vi "Relink Packages.vi"(8 "error in (no error)":errorcluster, 11 "Folders to relink":string[](array[string])) -> (0 "error out":errorcluster, 1 "Done":bool, 2 "report log out":string[](array[string]), 3 "Saved Items out":T1(array[cluster]))   [LabVIEW 2020]
doc: "Relinks LabVIEW packages after files were moved, generalising Relink Package.vi from one folder to an array of folders.\n\nTwo-phase design: Phase A (discovering) opens every .lvlib/.lvclass under each folder (loading makes LabVIEW relink moved dependencies), walks their descendants and opens every loose .vi/.ctl/.vim not owned by a library. Nothing is saved in Phase A and every reference is held open across all folders (warm object cache). Libraries and items are deduplicated globally across folders and packages. Work items are collected as ONE cluster array {Folder, Name, Type String, Path, ref} - each library's own item is appended AFTER its members, so members always save before their owning library. The ref field is a variant carrying the VI or Library refnum (To Variant when collecting, Variant To Data with the class picked by Type String when saving/closing). Null-ref filtering: Get All Descendents also returns non-VI project items whose 'VI Reference' property reads back a null (0) refnum WITHOUT an error, so a descendant becomes a work item only when its Type String is 'VI' AND the VI Reference read had no error AND the refnum passes Not A Number/Path/Refnum?. A library whose open or descendant walk fails is recorded in Saved Items out (Type String 'Library', status = TRUE), its reference is closed immediately and never enters the work-item array.\n\nPhase B (saving) saves EVERY work item unconditionally - there is deliberately no dirty gate. Rationale: LabVIEW resolves moved/stale subVI paths at load WITHOUT setting the VI Modifications Bitset (measured: a VI with dead absolute linker paths read bitset = 0), so gating on the bitset skips exactly the files whose linker table needs rewriting. Unconditional saving matches VIPM behaviour. A failing save never aborts the pass - it is recorded per item in Saved Items out (status = TRUE). All references are closed after Phase B and Done becomes TRUE only after the closes complete.\n\nVI-Server polling contract: the caller sets 'Folders to relink' and error in, runs the VI, and may poll Progress Phase ('discovering' then 'saving'), Progress Total, Progress Done and Progress Item while it runs. With an empty folder array the VI finishes immediately with Done = TRUE, empty reports and no error."
uses:
  a6c5ae95-22bd-4c75-b5e1-b7ef04b7ddf2.vi
  018dfcb9-4c8e-49be-be6d-b19c84c3ecea.vi
  f1460510-d6ef-45a5-b954-0afa6c603d40.vi
  0105af62-cf63-4b41-8393-fe647030f84d.vi
  a43e3b37-a8ff-4dec-b57d-d584032e0765.vi
panel:
  out "Progress Item":string
  out "Progress Done":i32
  out "Progress Total":i32
  out "Progress Phase":string
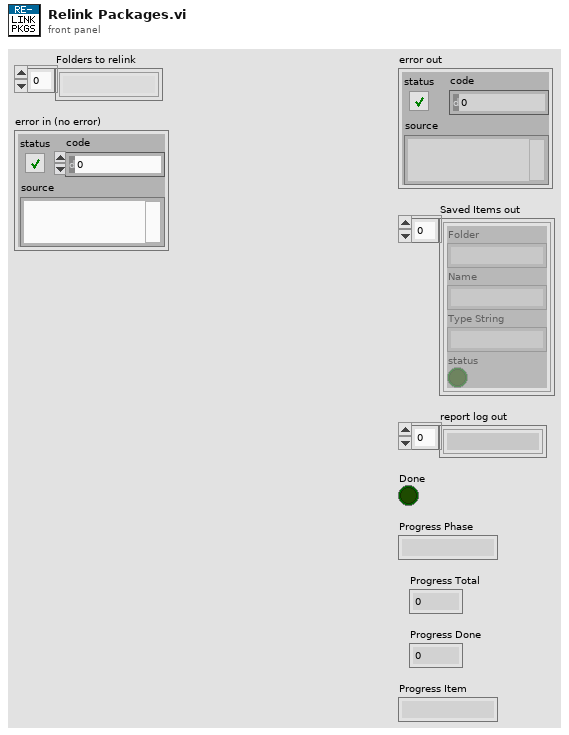
[diagram p1: front panel]
types:
  T1 = cluster{"Folder":string, "Name":string, "Type String":string, "status":bool}[]
  T2 = cluster{"Folder":string, "Name":string, "Type String":string, "Path":string, "ref":variant}[]
  T3 = cluster{"Folder":string, "Name":string, "Type String":string, "Path":string, "ref":variant}
  T4 = cluster{"Folder":string, "Name":string, "Type String":string, "status":bool}
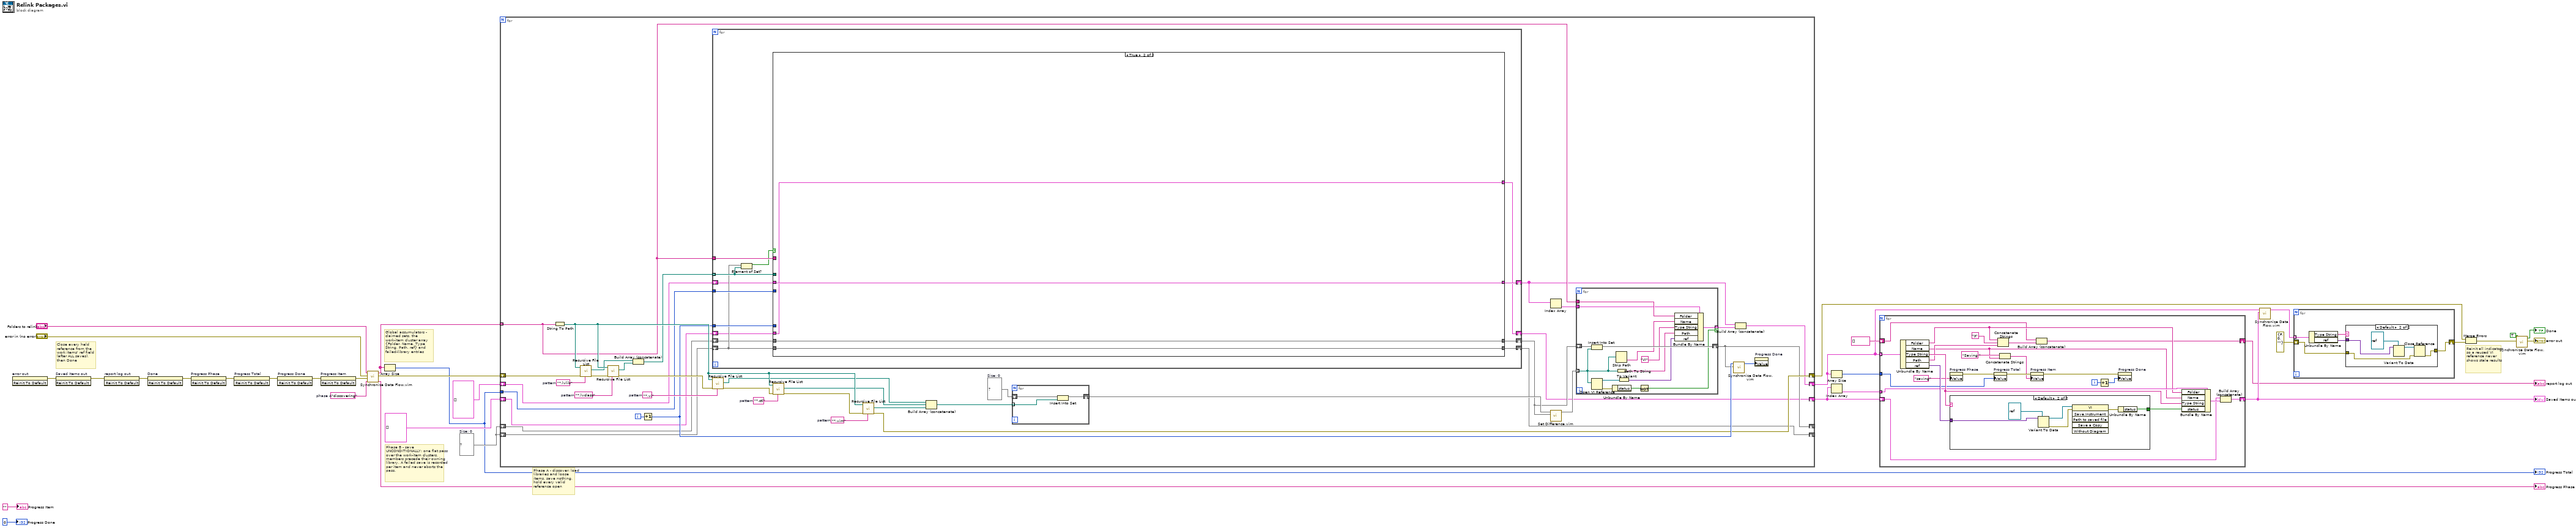
[diagram p0: block diagram]
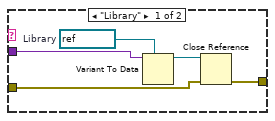
[diagram p2: hidden frame]
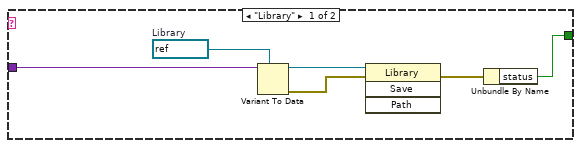
[diagram p3: hidden frame]
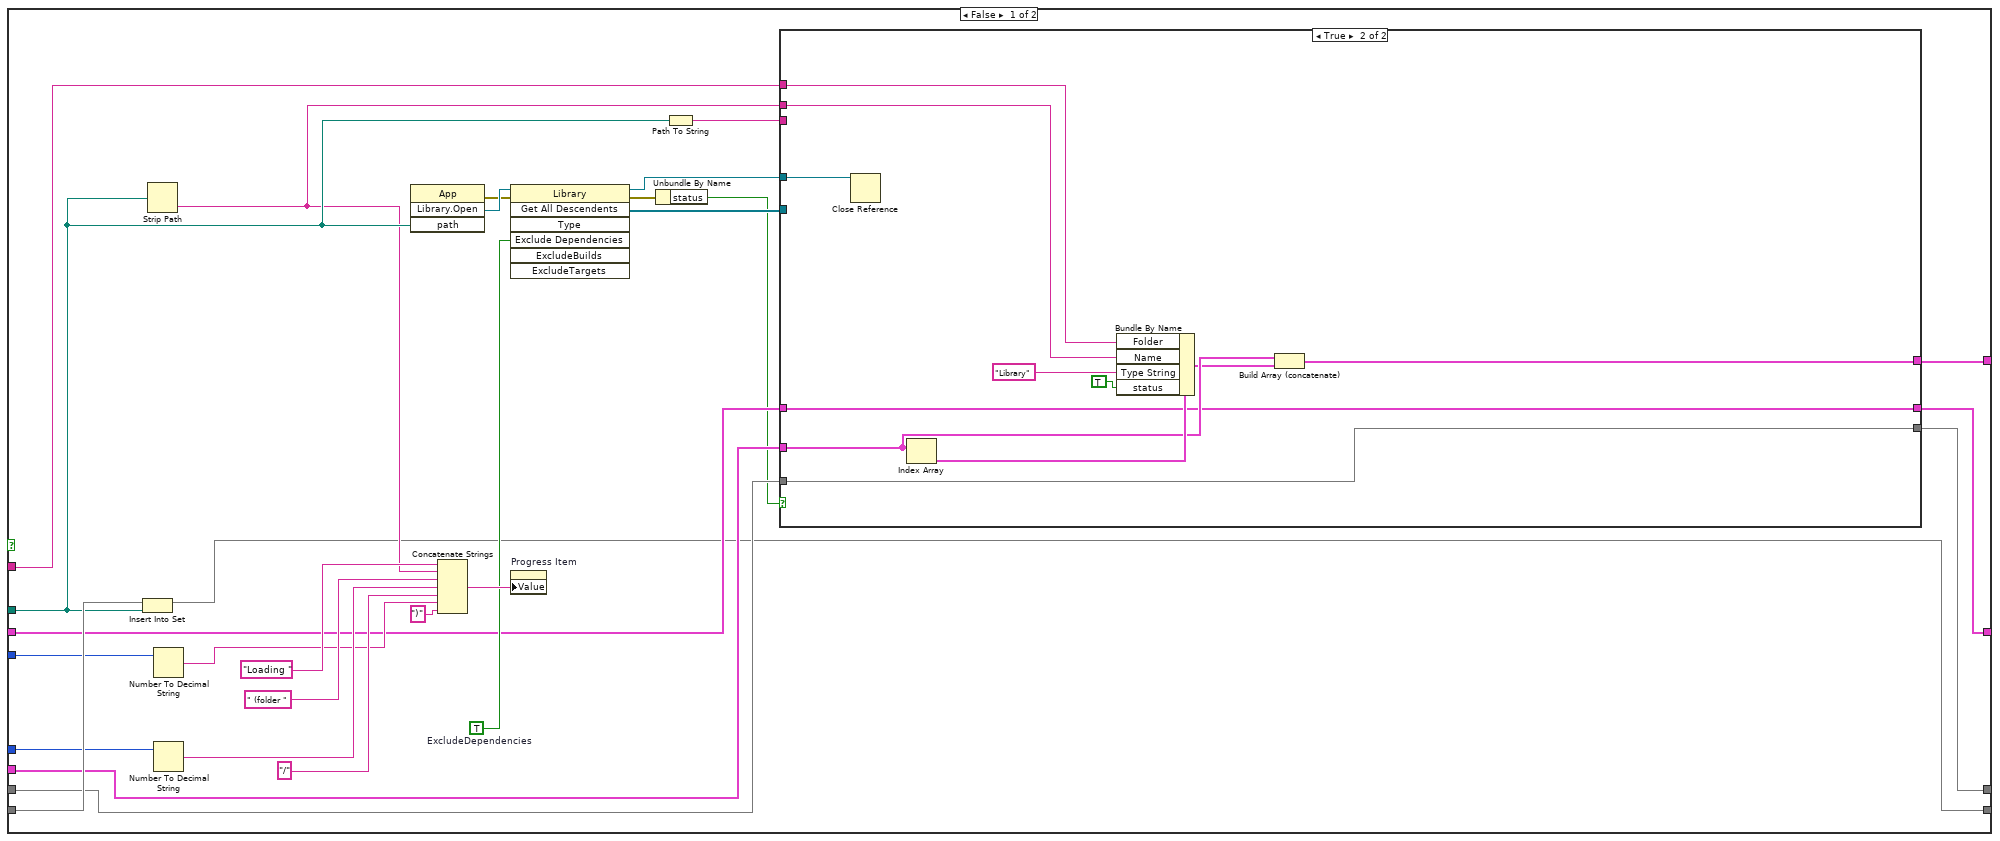
[diagram p4: hidden frame]
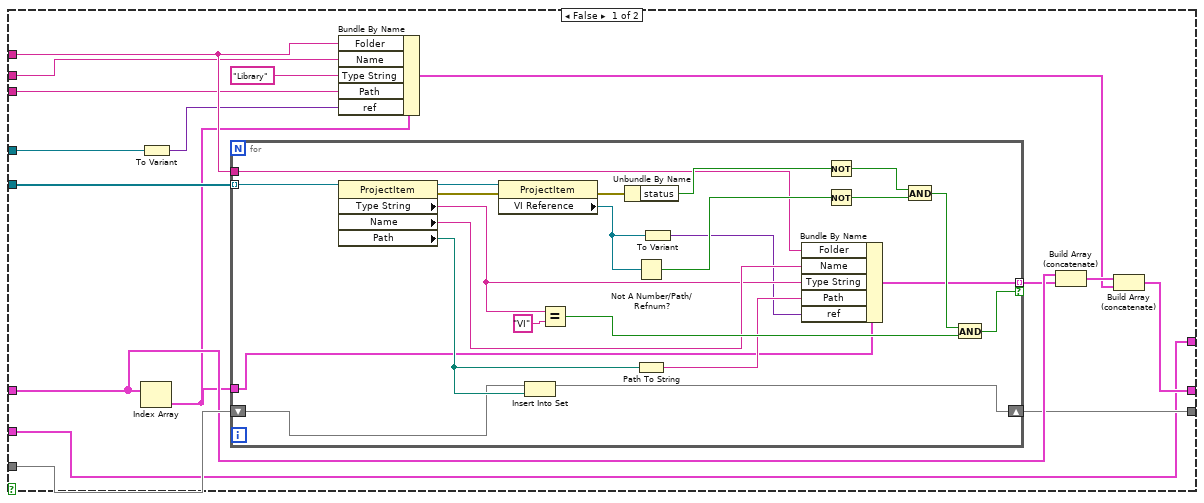
[diagram p5: hidden frame]
diagram:
  w22 = set{path} {}  # Size: 0
  w25 = "discovering"  # phase A
  # "Close every held reference from the work items' ref field (after ALL saves), then Done"
  # "Phase B - save UNCONDITIONALLY: one flat pass over the work-item clusters, members precede their owning library. A failed save is recorded per item and never aborts the pass."
  # "Phase A - discover: load libraries and loose items, save nothing, hold every valid reference open"
  # "Global accumulators - claimed sets, the work-item cluster array {Folder, Name, Type String, Path, ref} and failed-library entries"
  # "Reinit all indicators so a reused VI reference never shows stale results"
  n1 = invoke on="error out" class="Clust (strict)" method="Reinit To Default"() -> (error out=w35:errorcluster)  [unwired: 3 in, 2 out]
  n2 = invoke on="Saved Items out" class="Arr (strict)" method="Reinit To Default"(error in=w35) -> (error out=w34:errorcluster)  [unwired: 2 in, 2 out]
  n3 = invoke on="report log out" class="Arr (strict)" method="Reinit To Default"(error in=w34) -> (error out=w33:errorcluster)  [unwired: 2 in, 2 out]
  n4 = invoke on="Done" class="Bool (strict)" method="Reinit To Default"(error in=w33) -> (error out=w32:errorcluster)  [unwired: 2 in, 2 out]
  n5 = invoke on="Progress Phase" class="Str" method="Reinit To Default"(error in=w32) -> (error out=w31:errorcluster)  [unwired: 2 in, 2 out]
  n6 = invoke on="Progress Total" class="DigNum (strict)" method="Reinit To Default"(error in=w31) -> (error out=w30:errorcluster)  [unwired: 2 in, 2 out]
  n7 = invoke on="Progress Done" class="DigNum (strict)" method="Reinit To Default"(error in=w30) -> (error out=w29:errorcluster)  [unwired: 2 in, 2 out]
  n8 = invoke on="Progress Item" class="Str" method="Reinit To Default"(error in=w29) -> (error out=w26:errorcluster)  [unwired: 2 in, 2 out]
  n9 = call "Synchronize Data Flow.vim"("input 4"=w25, "input 3"=w26, "input 2"="error in (no error)", "input 1"="Folders to relink") -> ("output 4"=→"Progress Phase":string, "output 2"=w23:errorcluster, "output 1"=w24:string[])  [unwired: 1 out]
  n10 = Array Size(array=w24) -> (size(s)=w3:i32)
  "Progress Total" <- w3
  n11 = for {
    tunnel: w24 -> [w53] mode=indexing
    tunnel: w3 -> [w58]
    shift-right: [w46] -> w12
    shift-left: w23 -> [w45]
    shift-right: [w44] -> _
    shift-left: w22 -> [w43]
    shift-right: [w42] -> _
    shift-left: w22 -> [w41]
    shift-right: [w40] -> w15
    shift-left: T2 [] -> [w39]
    shift-right: [w38] -> w17
    shift-left: T1 [] -> [w37]
    i -> [w36]
    w56 = set{path} {}  # Size: 0
    w65 = "*.vim"  # pattern
    w68 = "*.ctl"  # pattern
    w70 = "*.vi"  # pattern
    w72 = "*.lvclass"  # pattern
    w74 = "*.lvlib"  # pattern
    n12 = String To Path(string=w53) -> (path=w67:path)
    n13 = call <vilib>:"Recursive File List.vi"("pattern"=w74, "error in (no error)"=w45, "Folder Path"=w67) -> ("error out"=w73:errorcluster, "All Files in Dir"=w64:path[])  [unwired: 4 in, 3 out]
    n14 = call <vilib>:"Recursive File List.vi"("pattern"=w72, "error in (no error)"=w73, "Folder Path"=w67) -> ("error out"=w71:errorcluster, "All Files in Dir"=w63:path[])  [unwired: 4 in, 3 out]
    n15 = Build Array (concatenate)(w64, w63) -> (w59:path[])
    n16 = Increment(x=w36) -> (x+1=w48:i32)
    n17 = for {
      tunnel: w59 -> [w104] mode=indexing
      tunnel: w53 -> [w103]
      tunnel: w48 -> [w102]
      tunnel: w58 -> [w101]
      shift-right: [w99] -> w44
      shift-left: w43 -> [w98]
      shift-right: [w97] -> w51
      shift-left: w41 -> [w96]
      shift-right: [w95] -> w50
      shift-left: w39 -> [w94]
      shift-right: [w93] -> w38
      shift-left: w37 -> [w92]
      n18 = Element of Set?(10:w104, 11:w98) -> (3:w100:bool)
      n19 = case shown="True" w100 {
        tunnel: w104 -> [w122 _]
        tunnel: w98 -> [w132 w186]
        tunnel: w96 -> [w115 w185]
        tunnel: w103 -> [w114 _]
        tunnel: w102 -> [w131 _]
        tunnel: w101 -> [w130 _]
        tunnel: w94 -> [w113 w184]
        tunnel: w92 -> [w112 w183]
        tunnel: [w108 w186] -> w99
        tunnel: [w107 w185] -> w97
        tunnel: [w106 w184] -> w95
        tunnel: [w105 w183] -> w93
        frame False {
          w119 = TRUE  # ExcludeDependencies
          n20 = Insert Into Set(10:w122, 11:w132) -> (3:w108:set{path})  [unwired: 1 out]
          n21 = Strip Path(path=w122) -> (name=w111:string)  [unwired: 1 out]
          n22 = Number To Decimal String(number=w130) -> (decimal integer string=w125:string)  [unwired: 1 in]
          n23 = Number To Decimal String(number=w131) -> (decimal integer string=w127:string)  [unwired: 1 in]
          n24 = invoke class="App" method="Library.Open"("path"=w122) -> (error out=w120:errorcluster, "Open Library"=w121:refnum<vi>)  [unwired: 3 in, 2 out]
          n25 = Concatenate Strings("Loading ", w111, " (folder ", w127, "/", w125, ")") -> (w123:string)
          n26 = invoke class="Library" method="Get All Descendents"(reference=w121, error in=w120, "Exclude Dependencies"=w119) -> (reference out=w116:refnum<vi>, error out=w118:errorcluster, "All Descendents"=w117:refnum<vi>[])  [unwired: 4 in, 4 out]
          n27 = property on="Progress Item" class="Str"("Value"=w123) -> ()  [unwired: 2 in, 2 out]
          n28 = Unbundle By Name(w118) -> ("status"=w109:bool)
          n29 = Path To String(path=w122) -> (string=w110:string)
          n30 = case shown="True" w109 {
            tunnel: w117 -> [w148 _]
            tunnel: w116 -> [w144 w182]
            tunnel: w115 -> [w147 w174]
            tunnel: w114 -> [w143 w181]
            tunnel: w113 -> [w146 w173]
            tunnel: w112 -> [w133 w176]
            tunnel: w111 -> [w142 w180]
            tunnel: w110 -> [w140 _]
            tunnel: [w135 w174] -> w107
            tunnel: [w134 w173] -> w106
            tunnel: [w133 w172] -> w105
            frame False {
              n31 = Index Array(array=w146) -> (element=w138:T3)  [unwired: 1 in]
              n32 = To Variant(anything=w144) -> (Variant=w139:variant)
              n33 = for {
                tunnel: w148 -> [w171] mode=indexing
                tunnel: w143 -> [w156]
                tunnel: w138 -> [w151]
                shift-right: [w159] -> w135
                shift-left: w147 -> [w158]
                tunnel: [w149] -> w145 mode=indexing if=w150
                n34 = property class="ProjectItem"(reference=w171) -> (reference out=w170:refnum<vi>, error out=w169:errorcluster, "Type String"=w154:string, "Name"=w155:string, "Path"=w160:path)  [unwired: 1 in]
                n35 = property class="ProjectItem"(reference=w170, error in=w169) -> (error out=w168:errorcluster, "VI Reference"=w157:refnum<vi>)  [unwired: 1 out]
                n36 = Insert Into Set(10:w160, 11:w158) -> (3:w159:set{path})  [unwired: 1 out]
                n37 = Equal?(x=w154, y="VI") -> (x = y?=w161:bool)
                n38 = Unbundle By Name(w168) -> ("status"=w167:bool)
                n39 = Not A Number/Path/Refnum?(number/path/refnum=w157) -> (NaN/Path/Refnum?=w166:bool)
                n40 = Path To String(path=w160) -> (string=w153:string)
                n41 = To Variant(anything=w157) -> (Variant=w152:variant)
                n42 = Bundle By Name(cluster=w151, "Folder"=w156, "Name"=w155, "Type String"=w154, "Path"=w153, "ref"=w152) -> (w149:T3)
                n43 = Not(x=w167) -> (.not. x?=w164:bool)
                n44 = Not(x=w166) -> (.not. x?=w163:bool)
                n45 = And(x=w164, y=w163) -> (x .and. y?=w162:bool)
                n46 = And(x=w162, y=w161) -> (x .and. y?=w150:bool)
              }
              n47 = Bundle By Name(cluster=w138, "Folder"=w143, "Name"=w142, "Type String"="Library", "Path"=w140, "ref"=w139) -> (w136:T3)
              n48 = Build Array (concatenate)(w146, w145) -> (w137:T2)
              n49 = Build Array (concatenate)(w137, w136) -> (w134:T2)
            }
            frame True {
              n50 = Close Reference(reference=w182) -> ()  [unwired: 1 in, 1 out]
              n51 = Index Array(array=w176) -> (element=w177:T4)  [unwired: 1 in]
              n52 = Bundle By Name(cluster=w177, "Folder"=w181, "Name"=w180, "Type String"="Library", "status"=TRUE) -> (w175:T4)
              n53 = Build Array (concatenate)(w176, w175) -> (w172:T1)
            }
          }
        }
        frame True {
        }
      }
    }
    n54 = call <vilib>:"Recursive File List.vi"("pattern"=w70, "error in (no error)"=w71, "Folder Path"=w67) -> ("error out"=w69:errorcluster, "All Files in Dir"=w62:path[])  [unwired: 4 in, 3 out]
    n55 = call <vilib>:"Recursive File List.vi"("pattern"=w68, "error in (no error)"=w69, "Folder Path"=w67) -> ("error out"=w66:errorcluster, "All Files in Dir"=w61:path[])  [unwired: 4 in, 3 out]
    n56 = call <vilib>:"Recursive File List.vi"("pattern"=w65, "error in (no error)"=w66, "Folder Path"=w67) -> ("error out"=w46:errorcluster, "All Files in Dir"=w60:path[])  [unwired: 4 in, 3 out]
    n57 = Build Array (concatenate)(w62, w61, w60) -> (w57:path[])
    n58 = for {
      tunnel: w57 -> [w91] mode=indexing
      shift-right: [w90] -> w55
      shift-left: w56 -> [w89]
      n59 = Insert Into Set(10:w91, 11:w89) -> (3:w90:set{path})  [unwired: 1 out]
    }
    n60 = Index Array(array=w50) -> (element=w52:T3)  [unwired: 1 in]
    n61 = call "Set Difference.vim"("set 2"=w51, "set 1"=w55) -> ("difference"=w54:set{path})  [unwired: 9 in]
    n62 = for {
      tunnel: w54 -> [w86] mode=indexing
      tunnel: w53 -> [w82]
      tunnel: w52 -> [w77]
      shift-right: [w85] -> w42
      shift-left: w51 -> [w84]
      tunnel: [w75] -> w49 mode=indexing if=w76
      n63 = Insert Into Set(10:w86, 11:w84) -> (3:w85:set{path})  [unwired: 1 out]
      n64 = Open VI Reference(vi path=w86) -> (vi reference=w83:refnum<vi>, error out=w88:errorcluster)  [unwired: 5 in]
      n65 = Unbundle By Name(w88) -> ("status"=w87:bool)
      n66 = Strip Path(path=w86) -> (name=w81:string)  [unwired: 1 out]
      n67 = Path To String(path=w86) -> (string=w79:string)
      n68 = To Variant(anything=w83) -> (Variant=w78:variant)
      n69 = Not(x=w87) -> (.not. x?=w76:bool)
      n70 = Bundle By Name(cluster=w77, "Folder"=w82, "Name"=w81, "Type String"="VI", "Path"=w79, "ref"=w78) -> (w75:T3)
    }
    n71 = call "Synchronize Data Flow.vim"("input 2"=w42, "input 1"=w48) -> ("output 1"=w47:i32)  [unwired: 2 in, 3 out]
    n72 = Build Array (concatenate)(w50, w49) -> (w40:T2)
    n73 = property on="Progress Done" class="DigNum (strict)"("Value"=w47) -> ()  [unwired: 2 in, 2 out]
  }
  n74 = Array Size(array=w15) -> (size(s)=w19:i32)
  n75 = Index Array(array=w17) -> (element=w18:T4)  [unwired: 1 in]
  n76 = for {
    tunnel: w15 -> [w210] mode=indexing
    tunnel: w19 -> [w198]
    tunnel: w18 -> [w206]
    shift-right: [w191] -> w7
    shift-left: w17 -> [w190]
    shift-right: [w189] -> w6
    shift-left: string[] [] -> [w188]
    i -> [w187]
    n77 = Unbundle By Name(w210) -> ("Folder"=w204:string, "Name"=w196:string, "Type String"=w208:string, "Path"=w202:string, "ref"=w209:variant)
    n78 = property on="Progress Phase" class="Str"("Value"="saving") -> (error out=w199:errorcluster)  [unwired: 2 in, 1 out]
    n79 = case shown="Default" w208 {
      tunnel: w209 -> [w216 w222]
      tunnel: [w211 w217] -> w207
      frame "Library" {
        w215 = refnum<vi> refnum  # Library
        n80 = Variant To Data(type=w215, Variant=w216) -> (data=w214:refnum<vi>, error out=w213:errorcluster)  [unwired: 1 in]
        n81 = invoke class="Library" method="Save"(reference=w214, error in=w213) -> (error out=w212:errorcluster)  [unwired: 2 in, 3 out]
        n82 = Unbundle By Name(w212) -> ("status"=w211:bool)
      }
      frame Default {
        n83 = Variant To Data(type=refnum<vi> refnum, Variant=w222) -> (data=w220:refnum<vi>, error out=w219:errorcluster)  [unwired: 1 in]
        n84 = invoke class="VI" method="Save.Instrument"(reference=w220, error in=w219) -> (error out=w218:errorcluster)  [unwired: 4 in, 5 out]
        n85 = Unbundle By Name(w218) -> ("status"=w217:bool)
      }
    }
    n86 = property on="Progress Total" class="DigNum (strict)"(error in=w199, "Value"=w198) -> (error out=w195:errorcluster)  [unwired: 1 in, 1 out]
    n87 = Concatenate Strings(w204, "\t", w202) -> (w201:string)
    n88 = Concatenate Strings("Saving ", w196) -> (w194:string)
    n89 = property on="Progress Item" class="Str"(error in=w195, "Value"=w194) -> (error out=w193:errorcluster)  [unwired: 1 in, 1 out]
    n90 = Build Array (concatenate)(w188, w201) -> (w189:string[])
    n91 = Increment(x=w187) -> (x+1=w192:i32)
    n92 = property on="Progress Done" class="DigNum (strict)"(error in=w193, "Value"=w192) -> ()  [unwired: 1 in, 2 out]
    n93 = Bundle By Name(cluster=w206, "Folder"=w204, "Name"=w196, "Type String"=w208, "status"=w207) -> (w205:T4)
    n94 = Build Array (concatenate)(w190, w205) -> (w191:T1)
  }
  "Saved Items out" <- w7
  "report log out" <- w6
  n95 = call "Synchronize Data Flow.vim"("input 2"=w7, "input 1"=w15) -> ("output 1"=w14:T2)  [unwired: 2 in, 3 out]
  n96 = for {
    tunnel: w14 -> [w227] mode=indexing
    shift-right: [w224] -> w11
    shift-left: errorcluster {"status"=FALSE, "code"=0, "source"=""} -> [w223]
    n97 = Unbundle By Name(w227) -> ("Type String"=w225:string, "ref"=w226:variant)
    n98 = case shown="Default" w225 {
      tunnel: w226 -> [w232 w237]
      tunnel: w223 -> [w229 w234]
      tunnel: [w228 w233] -> w224
      frame "Library" {
        w231 = refnum<vi> refnum  # Library
        n99 = Variant To Data(type=w231, Variant=w232) -> (data=w230:refnum<vi>)  [unwired: 1 in, 1 out]
        n100 = Close Reference(reference=w230, error in (no error)=w229) -> (error out=w228:errorcluster)
      }
      frame Default {
        n101 = Variant To Data(type=refnum<vi> refnum, Variant=w237) -> (data=w235:refnum<vi>)  [unwired: 1 in, 1 out]
        n102 = Close Reference(reference=w235, error in (no error)=w234) -> (error out=w233:errorcluster)
      }
    }
  }
  n103 = Merge Errors(w12, w11) -> (w9:errorcluster)
  n104 = call "Synchronize Data Flow.vim"("input 2"=w9, "input 1"=TRUE) -> ("output 2"=→"error out":errorcluster, "output 1"=→"Done":bool)  [unwired: 2 in, 2 out]
  "Progress Done" <- 0
  "Progress Item" <- ""
